vi "onTestDiscovery.vi"(8 "error in (no error)":errorcluster, 11 "Unit Tests for Runner in":refnum<class "Unit Tests for Runner.lvclass">) -> (0 "error out":errorcluster, 2 "Test VIs":path[](array[path]), 3 "Unit Tests for Runner out":refnum<class "Unit Tests for Runner.lvclass">)   [LabVIEW 2013, in "Unit Tests for Runner.lvclass"]
uses:
  Unit Tests for Runner.lvclass
  Unit Tests for Runner.lvclass/Unit Tests for Runner.ctl
  classes/Test Runner.Collection/Test Runner.Collection.lvclass
  classes/Test/Test.lvclass
  classes/Assert/Assert.lvclass
  classes/Test Runner/Test Runner.lvclass
panel:
  out "Pass?":bool
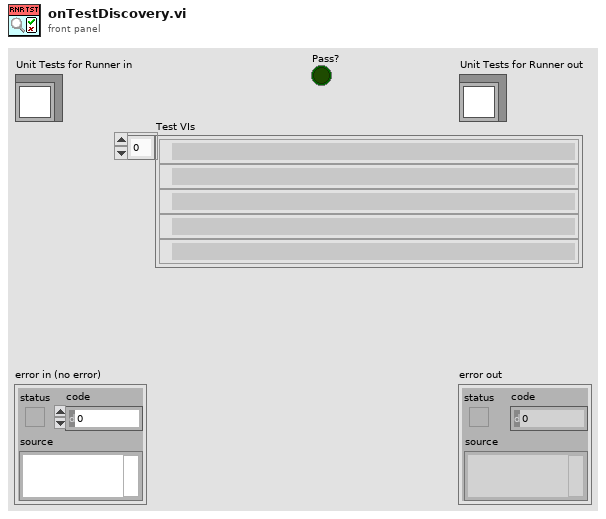
[diagram p1: front panel]
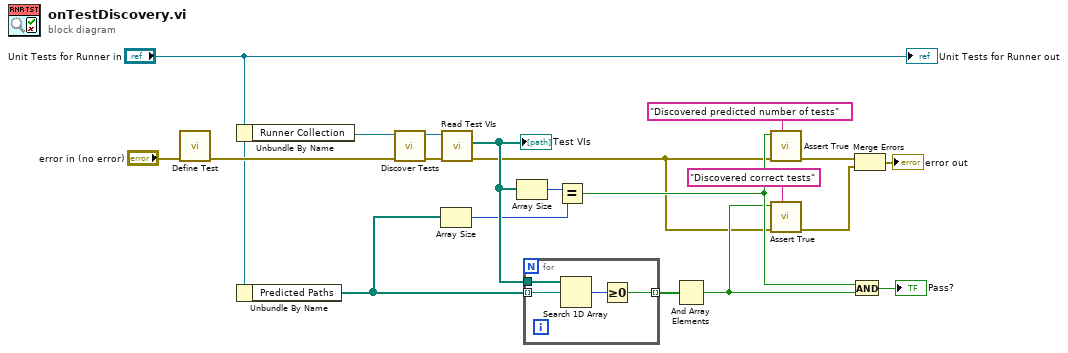
[diagram p0: block diagram]
diagram:
  n1 = call "Define Test.vi"("error in (no error)"="error in (no error)") -> ("error out"=w5:errorcluster)  [unwired: 10 in]
  n2 = Unbundle By Name("Unit Tests for Runner in") -> ("Runner Collection"=w6:refnum<class "Test Runner.Collection.lvclass">)
  n3 = Unbundle By Name("Unit Tests for Runner in") -> ("Predicted Paths"=w3:path[])
  n4 = call "Discover Tests.vi"("error in (no error)"=w5, "Test Runner in"=w6) -> ("error out"=w7:errorcluster, "Test Runner out"=w8:refnum<class "Test Runner.Collection.lvclass">)  [unwired: 8 in]
  n5 = Array Size(array=w3) -> (size(s)=w2:i32)
  n6 = call-dynamic "Read Test VIs.vi"("error in (no error)"=w7, "Test Runner in"=w8) -> ("error out"=w1:errorcluster, "Test VIs"=w11:path[])  [unwired: 7 in, 1 out]
  "Test VIs" <- w11
  n7 = Array Size(array=w11) -> (size(s)=w19:i32)
  n8 = for {
    tunnel: w11 -> [w24]
    tunnel: [w22] -> w10 mode=indexing
    tunnel: w3 -> [w21] mode=indexing
    n9 = Search 1D Array(1D array=w24, element=w21) -> (index of element=w23:i32)  [unwired: 1 in]
    n10 = Greater Or Equal To 0?(x=w23) -> (x >= 0?=w22:bool)
  }
  n11 = Equal?(x=w19, y=w2) -> (x = y?=w15:bool)
  n12 = And Array Elements(Boolean array=w10) -> (logical AND=w9:bool)
  n13 = call "Assert True.vi"("Label"="Discovered predicted number of tests", "error in (no error)"=w1, "True?"=w15) -> ("error out"=w18:errorcluster)  [unwired: 8 in]
  n14 = call "Assert True.vi"("Label"="Discovered correct tests", "error in (no error)"=w1, "True?"=w9) -> ("error out"=w17:errorcluster)  [unwired: 8 in]
  n15 = And(x=w15, y=w9) -> (x .and. y?=→"Pass?":bool)
  n16 = Merge Errors(w18, w17) -> (→"error out":errorcluster)
  "Unit Tests for Runner out" <- "Unit Tests for Runner in"
